vi "Output Sound Tone.vi"(5 "Time (s)":dbl=1.0, 6 "volume":dbl(slide)=100.0 min=0.0 max=100.0 step=1.0 scale=0.0..100.0, 7 "frequency":dbl=500.0 format="%0.2p", 8 "device ID":u32) -> (0 "error out":errorcluster)   [LabVIEW 2022 SP3]
uses:
  <vilib>/sound2/lvsound2.llb/Sound Data Format.ctl
  <vilib>/sound2/lvsound2.llb/Sampling Mode.ctl
  <vilib>/sound2/lvsound2.llb/Sound Output Set Volume (Single).vi
  <vilib>/sound2/lvsound2.llb/Sound Output Write (DBL Single).vi
  <vilib>/measure/NI_MABase.lvlib
panel:
  in  "sound format":T1={"sample rate (S/s)"=44100.0, "number of channels"=2, "bits per sample"=16}
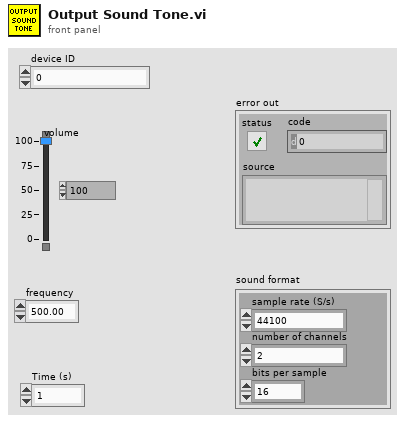
[diagram p1: front panel]
types:
  T1 = typedef "Sound Data Format.ctl" = cluster{"sample rate (S/s)":dbl, "number of channels":i32, "bits per sample":i32}
  T2 = typedef "Sampling Mode.ctl" = i32
  T3 = typedef "Sound Output Task ID.ctl" = u32
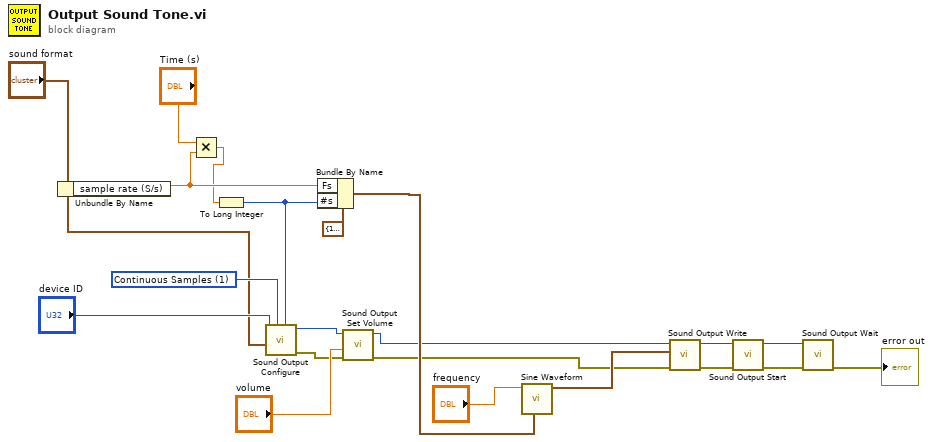
[diagram p0: block diagram]
diagram:
  w21 = T2 1 items=["Finite Samples", "Continuous Samples"] ("sample mode")
  n1 = Unbundle By Name("sound format") -> ("sample rate (S/s)"=w13:dbl)
  n2 = Multiply(x="Time (s)", y=w13) -> (x*y=w12:dbl)
  n3 = To Long Integer(number=w12) -> (32bit integer=w16:i32)
  n4 = call <vilib>:"Sound Output Configure.vi"("number of samples/ch"=w16, "sample mode"=w21, "sound format"="sound format", "device ID"="device ID") -> ("error out"=w2:errorcluster, "task ID"=w5:T3)  [unwired: 6 in]
  n5 = Bundle By Name(cluster=cluster{"Fs":dbl, "#s":dbl} {"Fs"=1000.0, "#s"=1000.0} ("sampling info"), "Fs"=w13, "#s"=w16) -> (w17:cluster{"Fs":dbl, "#s":dbl})
  n6 = call-poly <vilib>:"Sound Output Set Volume.vi"("error in (no error)"=w2, "volume"="volume", "task ID"=w5) -> ("error out"=w1:errorcluster, "task ID out"=w4:T3)  [unwired: 7 in]
  n7 = call <vilib>:"Sine Waveform.vi"("sampling info"=w17, "frequency"="frequency") -> ("signal out"=w7:waveform(dbl))  [unwired: 8 in, 1 out]
  n8 = call-poly <vilib>:"Sound Output Write.vi"("error in (no error)"=w1, "data"=w7, "task ID"=w4) -> ("error out"=w8:errorcluster, "task ID out"=w10:T3)  [unwired: 7 in]
  n9 = call <vilib>:"Sound Output Start.vi"("error in (no error)"=w8, "task ID"=w10) -> ("error out"=w9:errorcluster, "task ID out"=w11:T3)  [unwired: 8 in]
  n10 = call <vilib>:"Sound Output Wait.vi"("error in (no error)"=w9, "task ID"=w11) -> ("error out"=→"error out":errorcluster)  [unwired: 8 in, 1 out]
